vi "Lvi Set Trigger Threshold Channel.vi"(8 "error in (no error)":errorcluster, 10 "Channel":u32, 11 "TaskRef":i32) -> (0 "error out":errorcluster, 2 "function return":i32, 3 "TaskRef out":i32)   [LabVIEW 2022 SP3, in "DtLvLink.lvlib"]
doc: "Calls directly into the entry points of the DLL of the Data Acq SDK to specify which analog input channel to use for the threshold trigger for an analog input or analog output task. This VI is used by the higher-level VI, DtOLTrigger as well as the low-level VIs Lvi Set Trigger and Lvi Set Reference Trigger."
uses:
  DtLvLink.lvlib
  <userlib>/LV-Link3/DtLvLink_64.dll
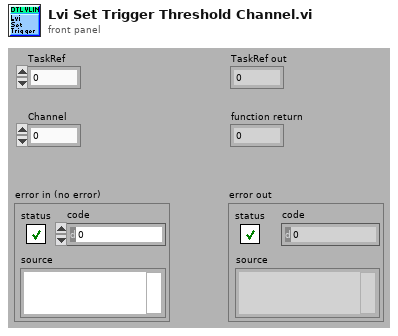
[diagram p1: front panel]
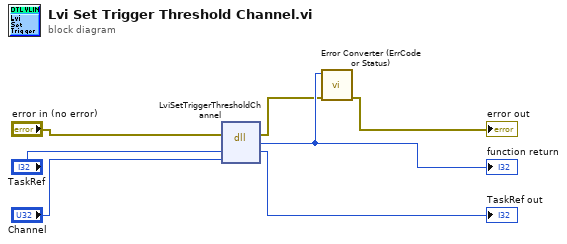
[diagram p0: block diagram]
diagram:
  n1 = dll-call lib="C:/Program Files/National Instruments/LabVIEW 2022/user.lib/LV-Link3/DtLvLink_64.*" fn="LviSetTriggerThresholdChannel"(error in="error in (no error)", "TaskRef"="TaskRef", "Channel"="Channel") -> (error out=w2:errorcluster, "return type"=w7:i32, "TaskRef"=→"TaskRef out":i32)  [unwired: 3 in, 1 out]
  "function return" <- w7
  n2 = call "Error Converter (ErrCode or Status).vi"("error in (no error)"=w2, "error code"=w7) -> ("error out"=→"error out":errorcluster)  [unwired: 9 in]
